vi "CPP-ZeroMaintenance.vi"(2 "Previous Scan Value":dbl, 3 "Ch Description":T2={"Ch Name"="Tunnel3:Pressures:", "Type"="", "Function"=enum."Analogue Input", "Ch State"=enum."On", "Calibration type"="", "A"=30.0, "B"=10.0, "C"=0.0, "D"=0.0, "Comments"="", "Address"={"Main"=0, "Ch."=0, "Sub"=0, "Port Name"=""}, "String"="", "Duty"=65535} {"Duty" format="%016b"; "D" format="%#_5g"; "C" format="%#_5g"; "B" format="%#_5g"; "A" format="%#_5g"}) -> (0 "Time Elapsed since zero (min)":dbl format="%#.2f", 1 "HelpText":string)   [LabVIEW 2016]
doc: "This VI performs the Auto Zeroing routine. All of the information for a given Rig should be included in the Channel Description for this to work correctly. The Channel name is not terribly important, but the assumed convention is < Rig Name >:Pressures:\n\nA := Seconds to Monitor is the interval used to determine whether the tunnel has been off long enough\nB := Seconds to Average is the averaging interval for recording zeroes\nC := timestamp of most recent Zero\nD := timestamp of previous Zero\n\nThe String element should be a semi-colon-separated array of ADAM Chs. The first Ch in the array should be the Listener Ch which is compared with the Threshold to determine if the tunnel is OFF. The remaining array of ADAM Chs should be all of the Pressure Chs that are to be auto-zeroed."
uses:
  ADAM Client/Sub VIs/ADAM Controls/Ch_description_ADAM.ctl
  ADAM Client/Sub VIs/ADAM Controls/Module_type_ADAM.ctl
  ADAM Client/Sub VIs/ADAM Controls/Function_ADAM.ctl
  ADAM Client/Sub VIs/ADAM Controls/Channel_State.ctl
  ADAM Client/Sub VIs/ADAM Controls/Calib_type_ADAM.ctl
  ADAM Client/Sub VIs/ADAM Controls/Address.ctl
panel:
  in  "Tab Control":T1(tab)
  out "Listener Threshold":dbl
  out "Fresh Data Available?":bool
  out "Do Zeroes?":bool
  out "Below Threshold?":bool
  out "Listening Ch":string[](array[string])
  out "Pressure Chs":string[](array[string])
  out "Listening Value":dbl=0.2694398123338766
  out "current time":timestamp=timestamp(3521053420.076362 s since 1904-01-01)
  out "Current Time (sec)":dbl=3521053420.076362 format="%#.0f"
  out "LastZeroedSS":dbl=3521053410.165856 format="%#.0f"
  in  "Throwback (s)":dbl=10.0 format="%#_13g"
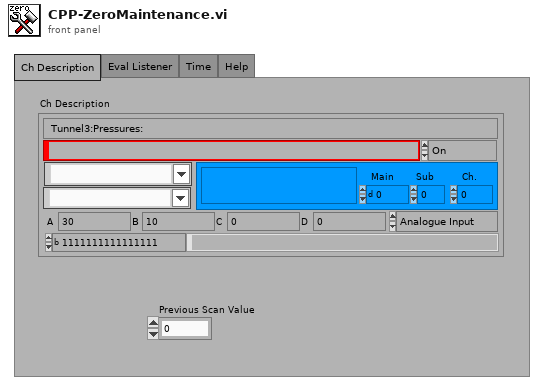
[diagram p1: front panel]
types:
  T1 = enum32{"Ch Description", "Eval Listener", "Time", "Help"}
  T2 = typedef "Ch_description_ADAM.ctl" = cluster{"Ch Name":string, "Type":T3, "Function":T4, "Ch State":T5, "Calibration type":T6, "A":dbl, "B":dbl, "C":dbl, "D":dbl, "Comments":string, "Address":T7, "String":string, "Duty":u16}
  T3 = typedef "Module_type_ADAM.ctl" = string
  T4 = typedef "Function_ADAM.ctl" = enum16{"Analogue Input", "Digital Input", "Event counter", "Event rate", "Analogue Output", "Digital Output", "Relay Output"}
  T5 = typedef "Channel_State.ctl" = enum16{"On", "Off", "Always On", "Always Off"}
  T6 = typedef "Calib_type_ADAM.ctl" = string
  T7 = typedef "Address.ctl" = cluster{"Main":i32, "Ch.":i32, "Sub":i32, "Port Name":string}
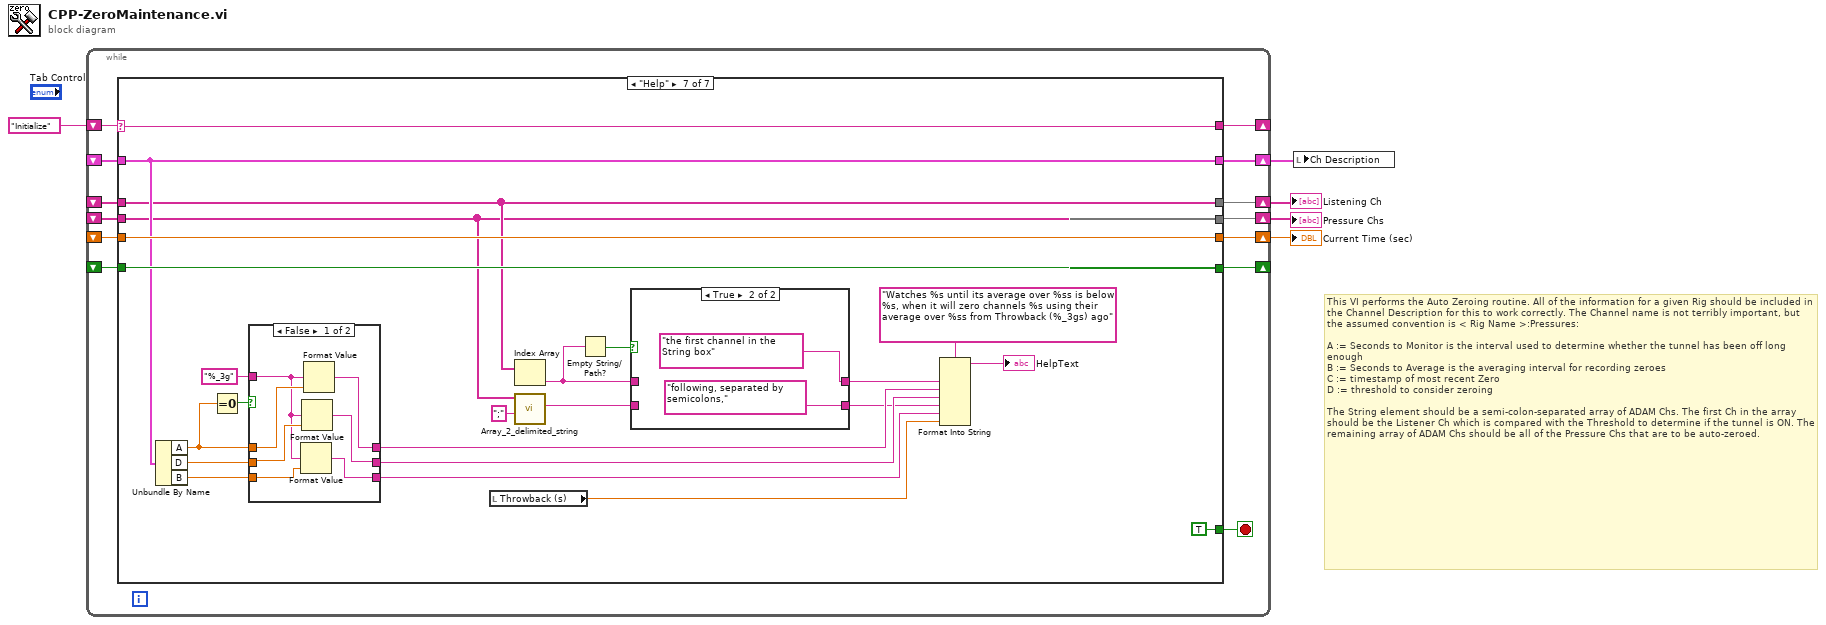
[diagram p0: block diagram]
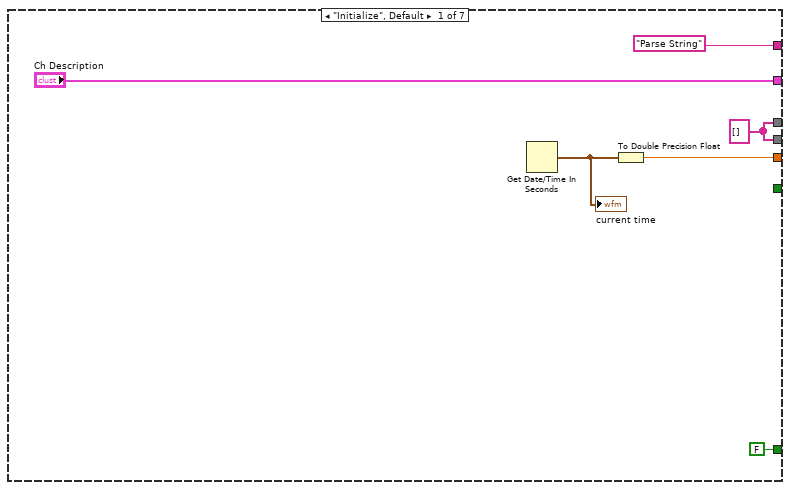
[diagram p2: hidden frame]
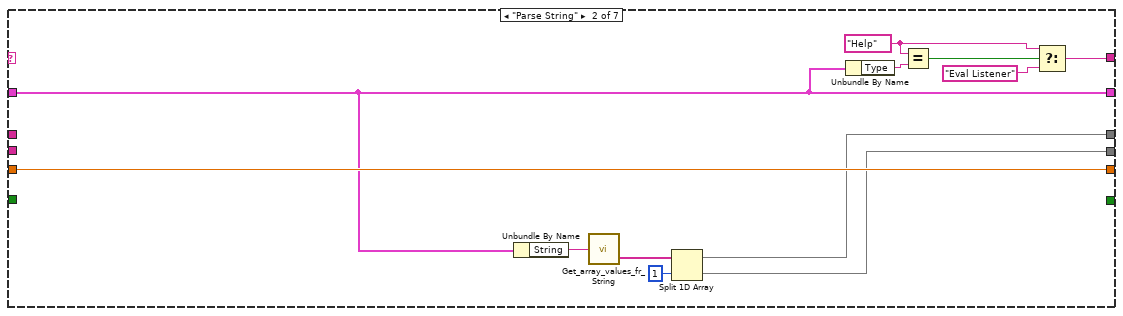
[diagram p3: hidden frame]
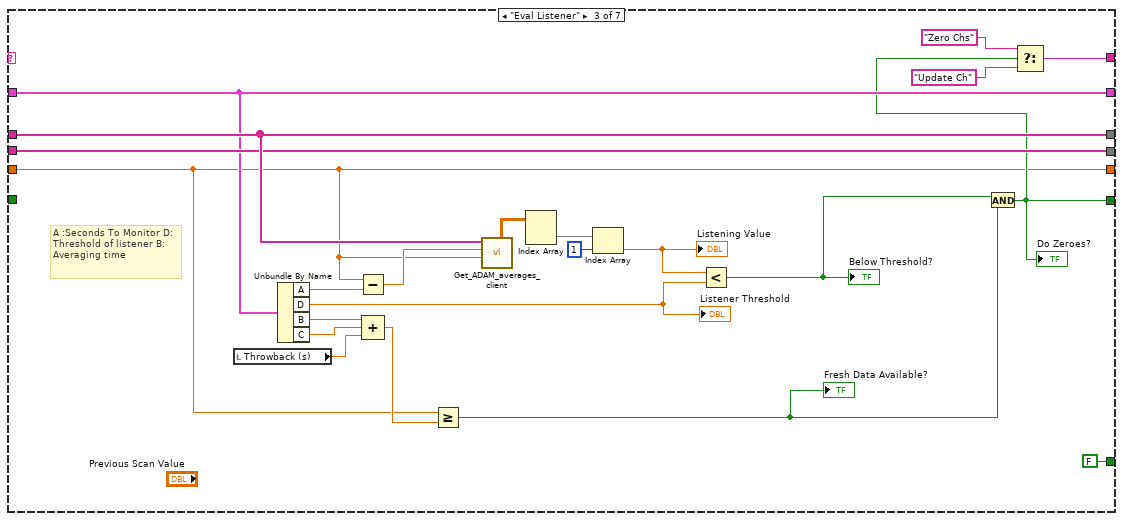
[diagram p4: hidden frame]
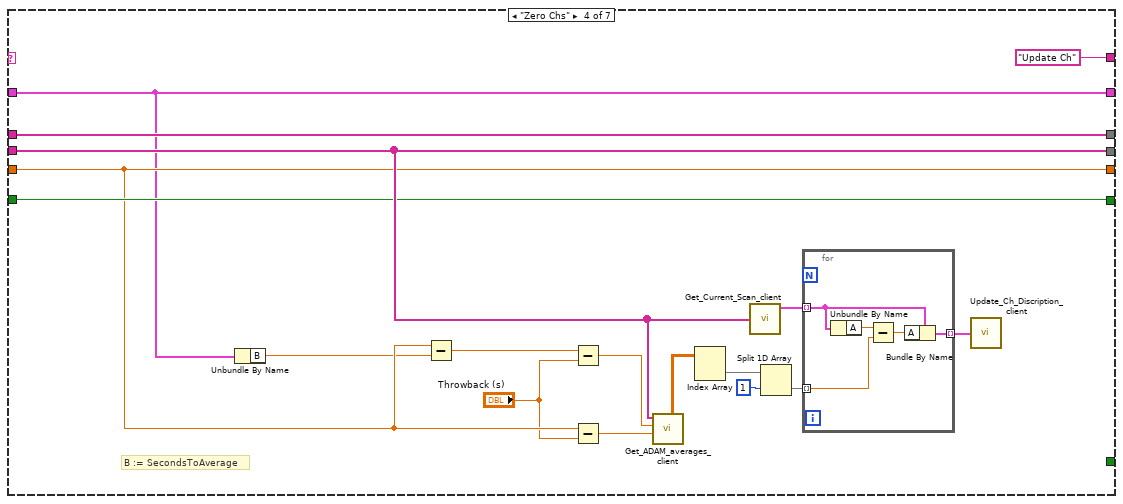
[diagram p5: hidden frame]
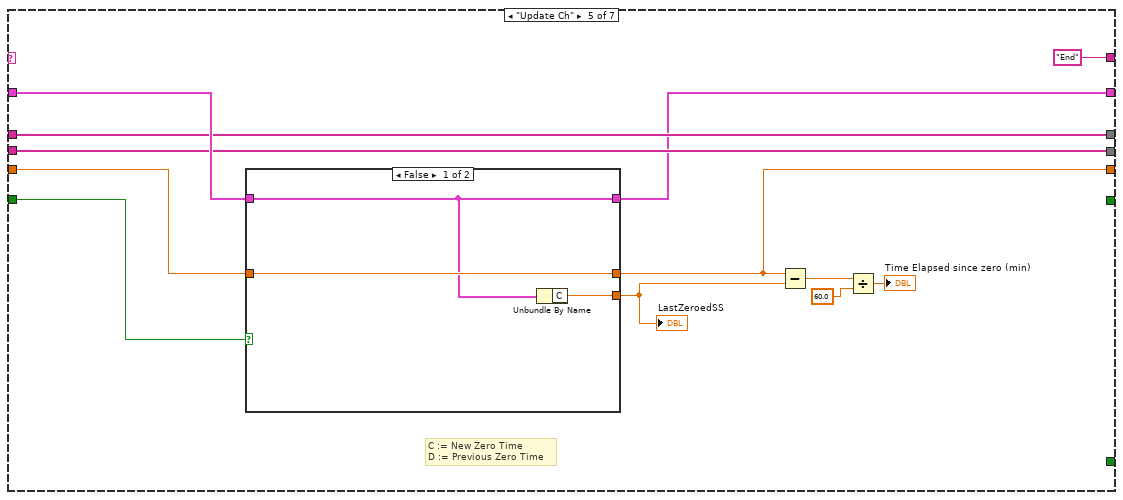
[diagram p6: hidden frame]
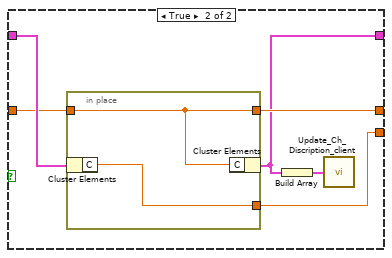
[diagram p7: hidden frame]
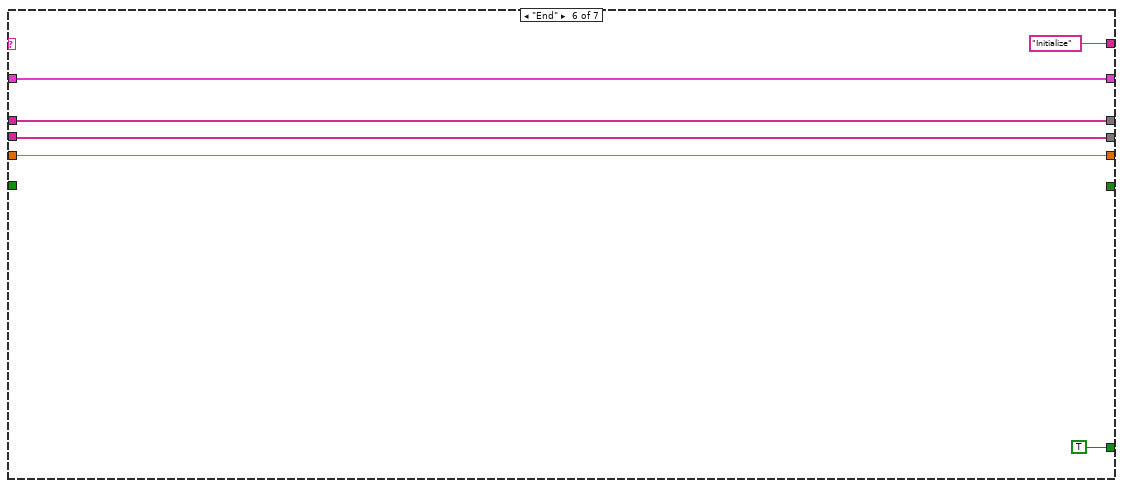
[diagram p8: hidden frame]
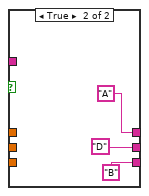
[diagram p10: hidden frame]
diagram:
  # "This VI performs the Auto Zeroing routine. All of the information for a given Rig should be included in the Channel Description for this to work correctly. The Channel name is not terribly important, but the assumed convention is < Rig Name >:Pressures:\n\nA := Seconds to Monitor is the interval used to determine whether the tunnel has been off long enough\nB := Seconds to Average is the averaging interval for recording zeroes\nC := timestamp of most recent Zero\nD := threshold to consider zeroing\n\nThe String element should be a semi-colon-separated array of ADAM Chs. The first Ch in the array should be the Listener Ch which is compared with the Threshold to determine if the tunnel is ON. The remaining array of ADAM Chs should be all of the Pressure Chs that are to be auto-zeroed."
  n1 = while {
    shift-right: [w17] -> _
    shift-left: "Initialize" -> [w18]
    shift-right: [w15] -> w1
    shift-left: _ -> [w16]
    shift-right: [w14] -> w3
    shift-left: _ -> [w13]
    shift-right: [w12] -> w2
    shift-left: _ -> [w11]
    shift-right: [w10] -> w4
    shift-left: _ -> [w8]
    shift-right: [w7] -> _
    shift-left: _ -> [w6]
    stop <- w9 stop-if-true
    n2 = case shown="\"Help\"" w18 {
      selector: w18 -> [_ _ _ _ _ _ w133]
      tunnel: ["Parse String" w27 w48 "Update Ch" "End" "Initialize" w133] -> w17
      tunnel: w16 -> [_ w26 w53 w70 w92 w108 w129]
      tunnel: ["Ch Description" w26 w53 w70 w82 w108 w129] -> w15
      tunnel: [w22 w32 w55 w74 w84 w106 w128] -> w14
      tunnel: w13 -> [_ _ w55 w74 w84 w106 w128]
      tunnel: [w22 w31 w54 w75 w83 w105 w124] -> w12
      tunnel: w11 -> [_ _ w54 w75 w83 w105 w124]
      tunnel: [w23 w35 w39 w71 w86 w104 w132] -> w10
      tunnel: [FALSE _ FALSE _ _ TRUE TRUE] -> w9
      tunnel: w8 -> [_ w35 w39 w71 w90 w104 w132]
      tunnel: [_ _ w42 w73 _ _ w131] -> w7
      tunnel: w6 -> [_ _ _ w73 w91 _ w131]
      frame "Initialize", Default {
        w22 = string[] []
        n3 = Get Date/Time In Seconds() -> (seconds since 1Jan1904=w24:timestamp)
        "current time" <- w24
        n4 = To Double Precision Float(number=w24) -> (double precision float=w23:dbl)
      }
      frame "Parse String" {
        w28 = T3 "Help" ("Type")
        n5 = Unbundle By Name(w26) -> ("String"=w36:string)
        n6 = call "Get_array_values_fr_String.vi"("String Value"=w36) -> ("String array"=w34:string[])  [unwired: 1 out]
        n7 = Split 1D Array(array=w34, index=1) -> (first subarray=w32:string[], second subarray=w31:string[])
        n8 = Unbundle By Name(w26) -> ("Type"=w25:T3)
        n9 = Equal?(x=w28, y=w25) -> (x = y?=w29:bool)
        n10 = Select(t=w28, s=w29, f="Eval Listener") -> (s? t:f=w27:T3)
      }
      frame "Eval Listener" {
        # "A :Seconds To Monitor D: Threshold of listener B: Averaging time"
        n11 = local read "Throwback (s)"() -> (w37:dbl)
        n12 = Unbundle By Name(w53) -> ("A"=w52:dbl, "D"=w40:dbl, "B"=w41:dbl, "C"=w38:dbl)
        "Listener Threshold" <- w40
        n13 = Subtract(x=w39, y=w52) -> (x-y=w56:dbl)
        n14 = Compound Arithmetic op=ADD(w41, w38, w37) -> (w44:dbl)
        n15 = Greater Or Equal?(x=w39, y=w44) -> (x >= y?=w45:bool)
        "Fresh Data Available?" <- w45
        n16 = call "Get_ADAM_averages_client.vi"("End time"=w39, "Start time"=w56, "ADAM Ch Names"=w55) -> ("DBL values"=w58:dbl[][])  [unwired: 4 in, 4 out]
        n17 = Index Array(array=w58) -> (element=w57:dbl[])  [unwired: 2 in]
        n18 = Index Array(array=w57, index=1) -> (element=w43:dbl)
        "Listening Value" <- w43
        n19 = Less?(x=w43, y=w40) -> (x < y?=w46:bool)
        "Below Threshold?" <- w46
        n20 = And(x=w46, y=w45) -> (x .and. y?=w42:bool)
        "Do Zeroes?" <- w42
        n21 = Select(t="Zero Chs", s=w42, f="Update Ch") -> (s? t:f=w48:string)
      }
      frame "Zero Chs" {
        # "B := SecondsToAverage"
        n22 = Unbundle By Name(w70) -> ("B"=w69:dbl)
        n23 = Subtract(x=w71, y=w69) -> (x-y=w65:dbl)
        n24 = Subtract(x=w65, y="Throwback (s)") -> (x-y=w66:dbl)
        n25 = Subtract(x=w71, y="Throwback (s)") -> (x-y=w67:dbl)
        n26 = call "Get_ADAM_averages_client.vi"("End time"=w67, "Start time"=w66, "ADAM Ch Names"=w75) -> ("DBL values"=w60:dbl[][])  [unwired: 4 in, 4 out]
        n27 = Index Array(array=w60) -> (element=w61:dbl[])  [unwired: 2 in]
        n28 = call "Get_Current_Scan_client.vi"("ADAM Ch Names"=w75) -> ("Ch Description Array"=w59:T2[])  [unwired: 3 out]
        n29 = Split 1D Array(array=w61, index=1) -> (second subarray=w62:dbl[])  [unwired: 1 out]
        n30 = for {
          tunnel: w59 -> [w78] mode=indexing
          tunnel: w62 -> [w79] mode=indexing
          tunnel: [w76] -> w64 mode=indexing
          n31 = Unbundle By Name(w78) -> ("A"=w80:dbl)
          n32 = Subtract(x=w80, y=w79) -> (x-y=w77:dbl)
          n33 = Bundle By Name(cluster=w78, "A"=w77) -> (w76:T2)
        }
        n34 = call "Update_Ch_Discription_client.vi"("Channels to update In"=w64) -> ()  [unwired: 1 out]
      }
      frame "Update Ch" {
        # "C := New Zero Time\nD := Previous Zero Time"
        n35 = case shown="False" w91 {
          tunnel: w92 -> [w94 w101]
          tunnel: w90 -> [w95 w100]
          tunnel: [w95 w97] -> w86
          tunnel: [w93 w98] -> w81
          tunnel: [w94 w96] -> w82
          frame False {
            n36 = Unbundle By Name(w94) -> ("C"=w93:dbl)
          }
          frame True {
            n37 = in-place {
              in-place-border: w100 -> [w103]
              in-place-border: [w103] -> w97
              in-place-border: [w102] -> w98
              n38 = in-place-cluster #1(w101) -> ("C"=w102:dbl)
              n39 = in-place-cluster #1("C"=w103) -> (w96:T2)
            }
            n40 = Build Array(w96) -> (w99:T2[])
            n41 = call "Update_Ch_Discription_client.vi"("Channels to update In"=w99) -> ()  [unwired: 1 out]
          }
        }
        "LastZeroedSS" <- w81
        n42 = Subtract(x=w86, y=w81) -> (x-y=w87:dbl)
        n43 = Divide(x=w87, y=60.0) -> (x/y=→"Time Elapsed since zero (min)":dbl)
      }
      frame "End" {
      }
      frame "Help" {
        n44 = Unbundle By Name(w129) -> ("A"=w120:dbl, "D"=w118:dbl, "B"=w116:dbl)
        n45 = Equal To 0?(x=w120) -> (x = 0?=w121:bool)
        n46 = case shown="False" w121 {
          tunnel: [w144 "A"] -> w122
          tunnel: w120 -> [w143 _]
          tunnel: [w141 "D"] -> w119
          tunnel: w118 -> [w142 _]
          tunnel: [w139 "B"] -> w117
          tunnel: w116 -> [w140 _]
          tunnel: "%_3g" ("format string") -> [w138 _]
          frame False {
            n47 = Format Value(format string=w138, value (0)=w140) -> (output string=w139:string)  [unwired: 1 in]
            n48 = Format Value(format string=w138, value (0)=w142) -> (output string=w141:string)  [unwired: 1 in]
            n49 = Format Value(format string=w138, value (0)=w143) -> (output string=w144:string)  [unwired: 1 in]
          }
          frame True {
          }
        }
        n50 = local read "Throwback (s)"() -> (w123:dbl)
        n51 = Index Array(array=w128) -> (element=w113:string)  [unwired: 1 in]
        n52 = call "Array_2_delimited_string.vi"("delimiter (Tab)"=";", "Array of Strings"=w124) -> ("delimited string"=w111:string)  [unwired: 9 in]
        n53 = Empty String/Path?(string/path=w113) -> (empty?=w110:bool)
        n54 = case shown="True" w110 {
          tunnel: [w135 "the first channel in the String box"] -> w114
          tunnel: w113 -> [w135 _]
          tunnel: [w134 "following, separated by semicolons," ("delimited string")] -> w112
          tunnel: w111 -> [w134 _]
          frame False {
          }
          frame True {
          }
        }
        n55 = Format Into String(format string="Watches %s until its average over %ss is below  %s, when it will zero channels %s using their average over %ss from Throwback (%_3gs) ago", w114, w122, w119, w112, w117, w123) -> (resulting string=→"HelpText":string)  [unwired: 2 in, 1 out]
      }
    }
  }
  "Current Time (sec)" <- w4
  "Listening Ch" <- w3
  "Pressure Chs" <- w2
  n56 = local write "Ch Description"(w1) -> ()
